vi "SeCrTs-DI waveform Samples bulider .vi"(7 "Samples":i32=10, 9 "Data input":waveform(dbl)[](array[waveform]), 11 "RD.DO_Data RD":refnum<queue>) -> (1 "Data out":waveform(dbl)[](array[waveform]))   [LabVIEW 2022 SP3]
panel:
  out "overflow?":bool
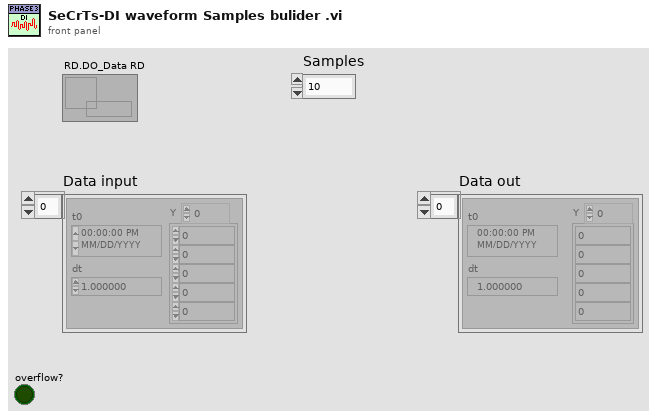
[diagram p1: front panel]
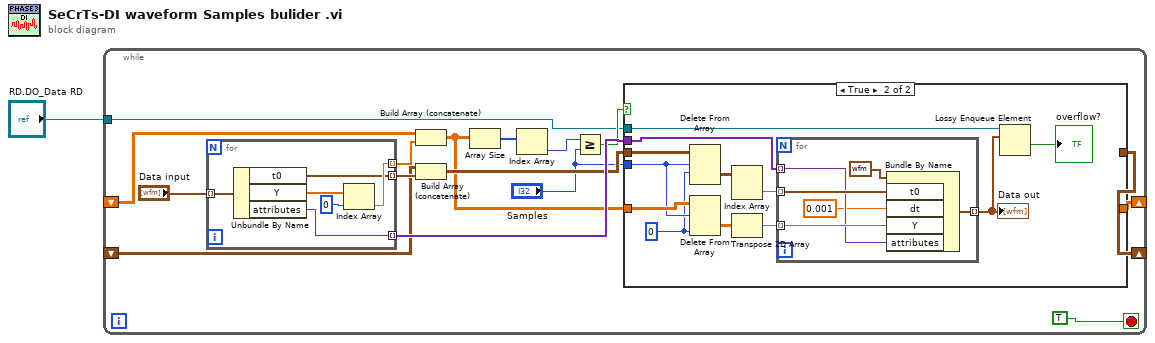
[diagram p0: block diagram]
diagram:
  n1 = while {
    shift-right: [w4] -> _
    shift-left: _ -> [w5]
    shift-right: [w3] -> _
    shift-left: _ -> [w6]
    tunnel: "RD.DO_Data RD" -> [w2]
    stop <- TRUE stop-if-true
    n2 = for {
      tunnel: "Data input" -> [w43] mode=indexing
      tunnel: [w41] -> w9 mode=indexing
      tunnel: [w39] -> w15 mode=indexing
      tunnel: [w38] -> w17 mode=indexing
      n3 = Unbundle By Name(w43) -> ("t0"=w39:timestamp, "Y"=w42:dbl[], "attributes"=w38:variant)
      n4 = Index Array(array=w42, index=0) -> (element=w41:dbl)
    }
    n5 = Build Array (concatenate)(w6, w9) -> (w12:dbl[][])
    n6 = Build Array (concatenate)(w5, w15) -> (w16:timestamp[][])
    n7 = Array Size(array=w12) -> (size(s)=w10:i32[])
    n8 = Index Array(array=w10) -> (element=w11:i32)  [unwired: 1 in]
    n9 = Greater Or Equal?(x=w11, y="Samples") -> (x >= y?=w13:bool)
    n10 = case shown="True" w13 {
      tunnel: w12 -> [w19 w31]
      tunnel: [w19 _] -> w3
      tunnel: w16 -> [w18 w29]
      tunnel: [w18 _] -> w4
      tunnel: w17 -> [_ w26]
      tunnel: "Samples" -> [_ w24]
      tunnel: w2 -> [_ w22]
      frame False {
      }
      frame True {
        w23 = 0 ("index (row)")
        n11 = Delete From Array(array=w29, length=w24, index (row)=w23) -> (deleted portion=w28:timestamp[][])  [unwired: 1 in, 1 out]
        n12 = Delete From Array(array=w31, length=w24, index (col)=w23) -> (deleted portion=w30:dbl[][])  [unwired: 1 in, 1 out]
        n13 = Index Array(array=w28) -> (element=w27:timestamp[])  [unwired: 2 in]
        n14 = Transpose 2D Array(2D array=w30) -> (transposed array=w25:dbl[][])
        n15 = for {
          tunnel: w25 -> [w37] mode=indexing
          tunnel: w27 -> [w36] mode=indexing
          tunnel: w26 -> [w35] mode=indexing
          tunnel: [w34] -> w21 mode=indexing
          n16 = Bundle By Name(cluster=waveform(dbl) {"t0"=timestamp(0 s since 1904-01-01), "dt"=1.0, "Y"=[]} ("output waveform"), "t0"=w36, "dt"=0.001, "Y"=w37, "attributes"=w35) -> (w34:waveform(dbl))
        }
        "Data out" <- w21
        n17 = Lossy Enqueue Element(queue=w22, element=w21) -> (overflow?=→"overflow?":bool)  [unwired: 1 in, 3 out]
      }
    }
  }
